vi "Get Preset Frequency Range.vi"(8 "error in (no error)":errorcluster {"code" format="%.0x"}, 11 "instrument handle":refnum<k15>) -> (0 "error out":errorcluster {"code" format="%.0x"}, 1 "MaxFreq":dbl, 2 "MinFreq":dbl, 3 "instrument handle out":refnum<k15>)   [LabVIEW 2014, in "Agilent NA.lvlib"]
doc: "Returns the preset frequencies range of the instrument."
uses:
  Agilent NA.lvlib
  AgNA.dll
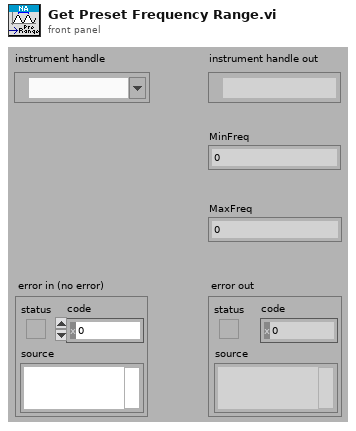
[diagram p1: front panel]
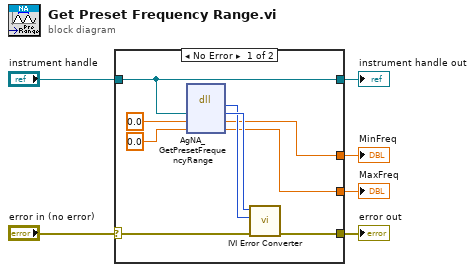
[diagram p0: block diagram]
diagram:
  n1 = case shown="No Error" "error in (no error)" {
    selector: "error in (no error)" -> [w13 w17]
    tunnel: [w12 w17] -> w6
    tunnel: [w10 _] -> w4
    tunnel: [w8 _] -> w3
    tunnel: [w7 w16] -> w2
    tunnel: "instrument handle" -> [w7 w16]
    frame No Error {
      n2 = dll-call lib="AgNA**.dll" fn="AgNA_GetPresetFrequencyRange"("Vi"=w7, "MinFreq"=0.0, "MaxFreq"=0.0) -> (w14:i32, "Vi"=w15:u32, "MinFreq"=w10:dbl, "MaxFreq"=w8:dbl)  [unwired: 3 in, 2 out]
      n3 = call "IVI Error Converter.vi"("error in (no error)"=w13, "IVI error code (0)"=w14, "instrument handle"=w15) -> ("error out"=w12:errorcluster)  [unwired: 7 in, 1 out]
    }
    frame Error {
    }
  }
  "error out" <- w6
  "instrument handle out" <- w2
  "MinFreq" <- w4
  "MaxFreq" <- w3
